vi "opencvSegment.vi"(0 "ImgIn":u16[](array[numeric]), 1 "sizex":i32, 2 "sizey":i32, 3 "ArrA":u16[](array[numeric]), 4 "ArrB":sgl[](array[numeric]), 5 "ArrBX":sgl[](array[numeric]), 6 "ArrBY":sgl[](array[numeric]), 7 "ArrBth":sgl[](array[numeric]), 8 "maxXInStack":dbl=1.0, 9 "ArrBdil":sgl[](array[numeric]), 10 "maxYInStack":dbl, 11 "ArrUno":sgl[](array[numeric]), 12 "threshold":sgl=0.25, 13 "NeuronXY":u16[](array[numeric]), 15 "NeuronN":u16) -> (14 "maxY":dbl, 16 "maxX":dbl, 18 "ArrA Out":u16[](array[numeric]), 20 "ArrB Out":sgl[](array[numeric]), 21 "ArrBX Out":sgl[](array[numeric]), 22 "ArrBY Out":sgl[](array[numeric]), 23 "ArrBth Out":sgl[](array[numeric]), 24 "ArrBdil Out":sgl[](array[numeric]), 25 "ArrUno Out":sgl[](array[numeric]), 26 "NeuronXY Out":u16[](array[numeric]), 27 "NeuronN Out":u16)   [LabVIEW 2017]
uses:
  dll/wormUtilities/x64/Release/wormUtilities.dll
panel:
  # "0.25"
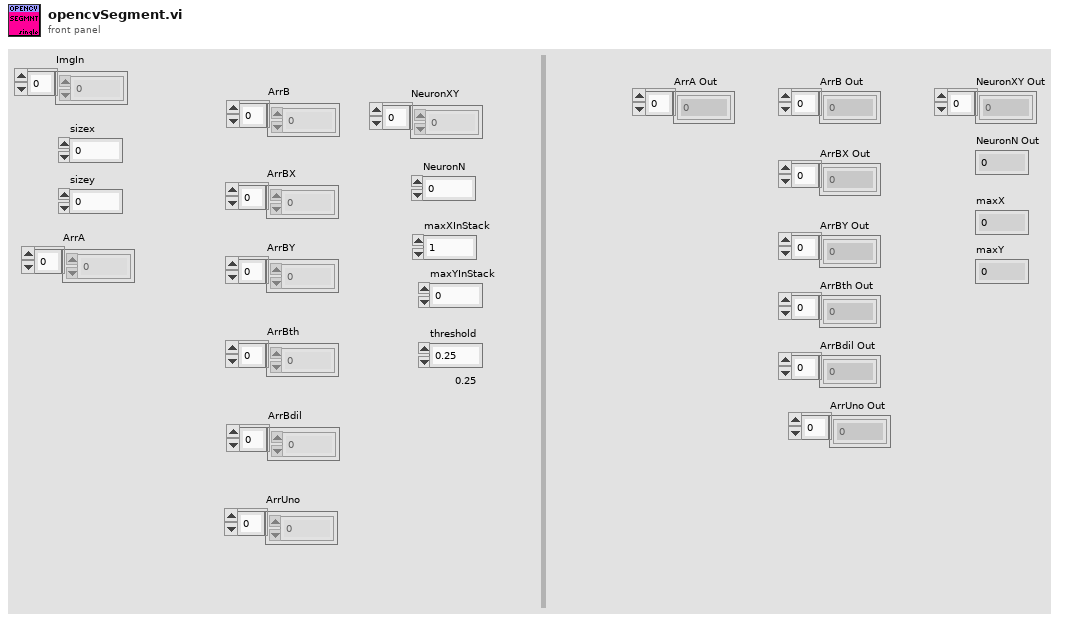
[diagram p1: front panel]
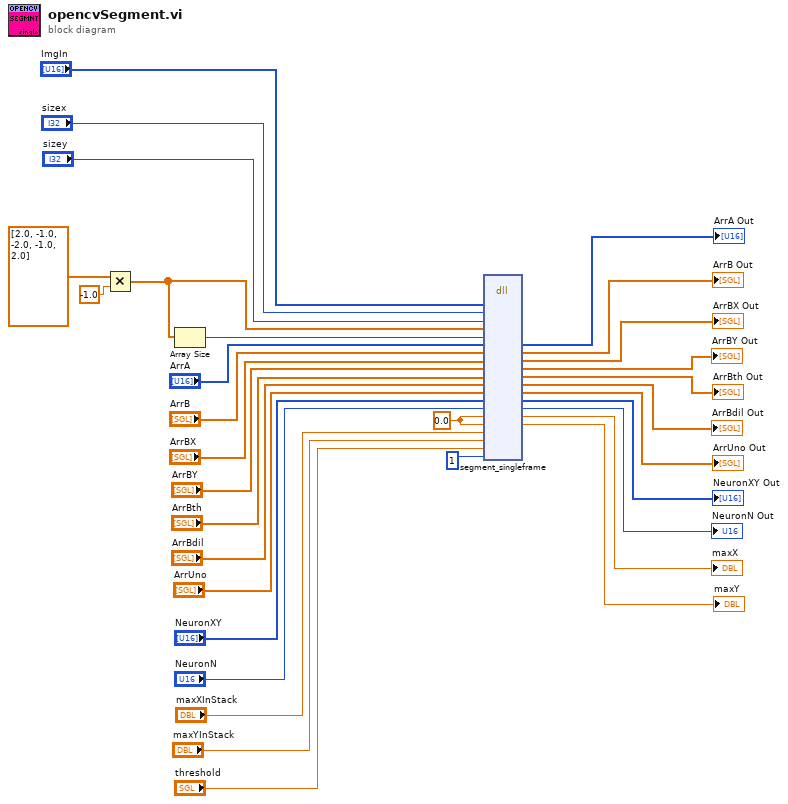
[diagram p0: block diagram]
diagram:
  w4 = 0.0 ("maxBXY")
  n1 = Multiply(x=sgl[] [2.0, -1.0, -2.0, -1.0, 2.0], y=sgl -1.0) -> (x*y=w30:sgl[])
  n2 = Array Size(array=w30) -> (size(s)=w29:i32)
  n3 = dll-call lib="C:/Users/francesco/dev/pump-probe/dll/wormUtilities/x64/Release/wormUtilities.dll" fn="segment_singleframe"("ImgIn"="ImgIn", "sizex"="sizex", "sizey"="sizey", "arrC"=w30, "sizeC"=w29, "ArrA"="ArrA", "ArrB"="ArrB", "ArrBX"="ArrBX", "ArrBY"="ArrBY", "ArrBth"="ArrBth", "ArrBdil"="ArrBdil", "ArrUno"="ArrUno", "NeuronXY"="NeuronXY", "NeuronN"="NeuronN", "maxX"=w4, "maxY"=w4, "maxXInStack"="maxXInStack", "maxYInStack"="maxYInStack", "threshold"="threshold", "resize"=i8 1) -> ("ArrA"=→"ArrA Out":u16[], "ArrB"=→"ArrB Out":sgl[], "ArrBX"=→"ArrBX Out":sgl[], "ArrBY"=→"ArrBY Out":sgl[], "ArrBth"=→"ArrBth Out":sgl[], "ArrBdil"=→"ArrBdil Out":sgl[], "ArrUno"=→"ArrUno Out":sgl[], "NeuronXY"=→"NeuronXY Out":u16[], "NeuronN"=→"NeuronN Out":u16, "maxX"=→"maxX":dbl, "maxY"=→"maxY":dbl)  [unwired: 13 in, 2 out]
